vi "Open TDMS.vi"(7 "Operation (1: open or create)":T1(ring)=enum."open or create", 8 "error in (no error)":errorcluster, 9 "Group":string, 10 "File Path":path, 11 "Parallax PING))) in":refnum<class "Parallax PING))).lvclass">) -> (0 "error out":errorcluster, 3 "Parallax PING))) out":refnum<class "Parallax PING))).lvclass">)   [LabVIEW 2013, in "Parallax PING))).lvclass"]
doc: "Opens a tdms file to record sensor data."
uses:
  Parallax PING))).lvclass
  Parallax PING))).lvclass/Parallax PING))).ctl
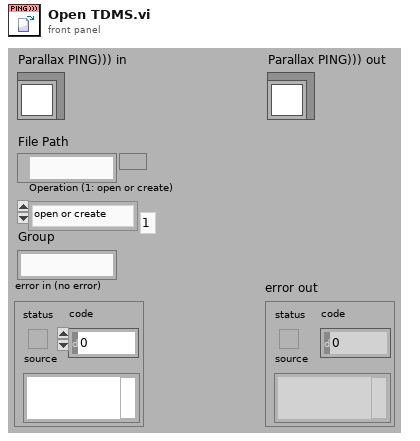
[diagram p1: front panel]
types:
  T1 = enum16{"open", "open or create", "create or replace", "create"}
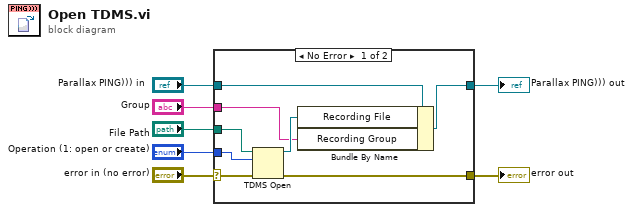
[diagram p0: block diagram]
diagram:
  n1 = case shown="No Error" "error in (no error)" {
    selector: "error in (no error)" -> [w15 w17]
    tunnel: [w8 w17] -> w6
    tunnel: [w9 w16] -> w4
    tunnel: "Parallax PING))) in" -> [w12 w16]
    tunnel: "File Path" -> [w14 _]
    tunnel: "Operation (1: open or create)" -> [w13 _]
    tunnel: "Group" -> [w10 _]
    frame No Error {
      n2 = TDMS Open(8:w15, 10:w13, 11:w14) -> (0:w8:errorcluster, 3:w11:refnum<k34>)  [unwired: 4 in]
      n3 = Bundle By Name(cluster=w12, "Recording File"=w11, "Recording Group"=w10) -> (w9:refnum<class "Parallax PING))).lvclass">)
    }
    frame Error {
    }
  }
  "error out" <- w6
  "Parallax PING))) out" <- w4
